vi "公式复合写入.vi"(8 "公式":cluster{"X^2":dbl, "X":dbl, "b":dbl}, 9 "量程下拉列表":enum16{"低量程", "高量程"}(ring), 10 "测量模式下拉列表":enum16{"水样测量", "零点核查", "跨度核查", "标样核查", "加标回收"}(ring), 11 "参数下拉列表":enum16{"COD", "氨氮", "总氮", "总磷"}(ring)) -> (3 "模型复制":T1)   [LabVIEW 2016, in "斯坦道氨氮.lvlib"]
uses:
  <vilib>/Utility/miscctls.llb/LVPointTypeDef.ctl
panel:
  out "连接的字符串":string
  in  "取消":bool
  in  "确认":bool
  in  "加标回收":bool
  in  "标样核查":bool
  in  "跨度核查":bool
  in  "空白核查":bool
  in  "水样测量":bool=TRUE
  # "请选择要写入的参数"
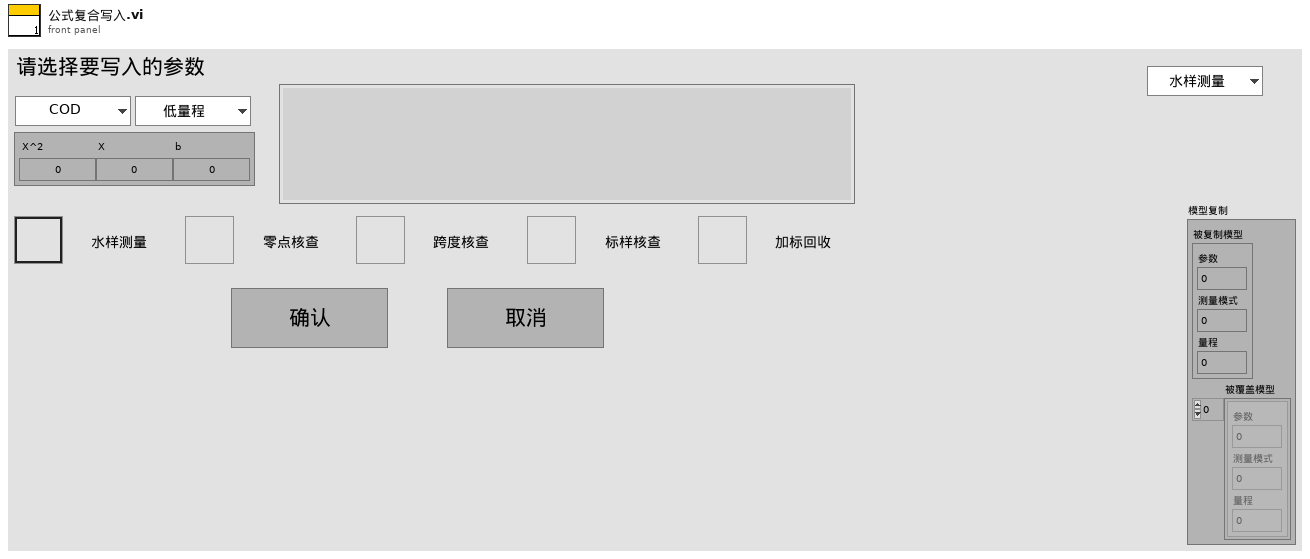
[diagram p1: front panel]
types:
  T1 = cluster{"被复制模型":cluster{"参数":u8, "测量模式":u8, "量程":u8}, "被覆盖模型":cluster{"参数":u8, "测量模式":u8, "量程":u8}[]}
  T2 = typedef "LVPointTypeDef.ctl" = cluster{"Horizontal":i16, "Vertical":i16}
  T3 = cluster{"COD":bool, "氨氮":bool, "总氮":bool, "总磷":bool}
  T4 = cluster{"测量量程":dbl, "测量精度":dbl, "测量间隔":dbl, "消解温度":dbl, "消解时长":dbl, "空白校准时间":timestamp, "曲线截距":dbl, "曲线斜率":dbl, "测量检出限":dbl, "测量信号值":dbl, "线性相关系数":dbl, "二次多项式系数":dbl, "标样校准时间":timestamp, "稀释倍数":dbl, "三项式系数":dbl, "空白标定系数":dbl, "量程系数":dbl, "F0/ORPA":dbl, "F1/ORPB":dbl, "F2/ORPK":dbl, "F3":dbl, "F4":dbl, "F5":dbl, "F6":dbl, "F7":dbl, "X0/滴定数":dbl, "量程":dbl}
  T5 = cluster{"参数下拉列表":enum16{"COD", "氨氮", "总氮", "总磷"}, "测量模式":enum16{"水样测量", "零点核查", "跨度核查", "标样核查", "加标回收"}, "量程下拉列表":enum16{"低量程", "高量程"}}
  T6 = cluster{"参数下拉列表":enum16{"COD", "氨氮", "总氮", "总磷"}, "测量模式":enum16{"水样测量", "零点核查", "跨度核查", "标样核查", "加标回收"}, "量程下拉列表":enum16{"低量程", "高量程"}}[]
  T7 = cluster{"参数下拉列表":enum16{"COD", "氨氮", "总氮", "总磷"}, "测量模式下拉列表":enum16{"水样测量", "零点核查", "跨度核查", "标样核查", "加标回收"}, "量程下拉列表":enum16{"低量程", "高量程"}}
  T8 = cluster{cluster{"参数下拉列表":enum16{"COD", "氨氮", "总氮", "总磷"}, "测量模式下拉列表":enum16{"水样测量", "零点核查", "跨度核查", "标样核查", "加标回收"}, "量程下拉列表":enum16{"低量程", "高量程"}}, cluster{"参数下拉列表":enum16{"COD", "氨氮", "总氮", "总磷"}, "测量模式下拉列表":enum16{"水样测量", "零点核查", "跨度核查", "标样核查", "加标回收"}, "量程下拉列表":enum16{"低量程", "高量程"}}[]}
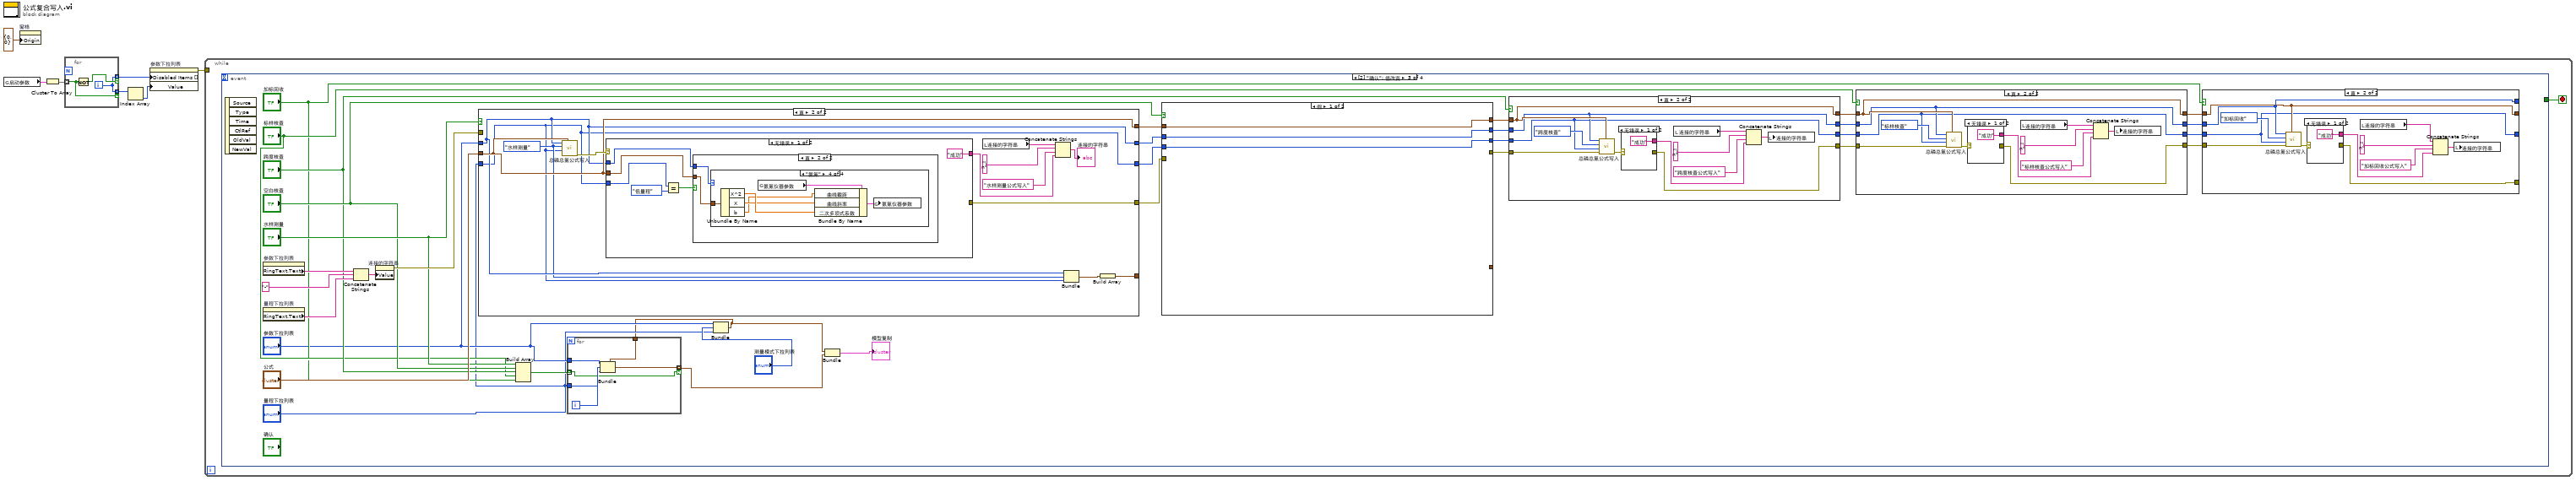
[diagram p0: block diagram]
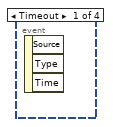
[diagram p2: hidden frame]
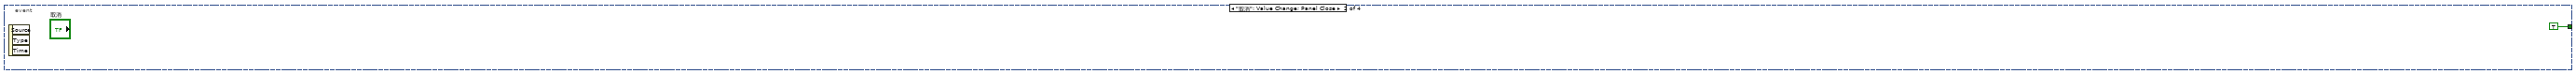
[diagram p3: hidden frame]
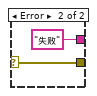
[diagram p5: hidden frame]
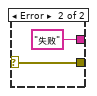
[diagram p7: hidden frame]
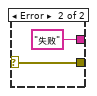
[diagram p9: hidden frame]
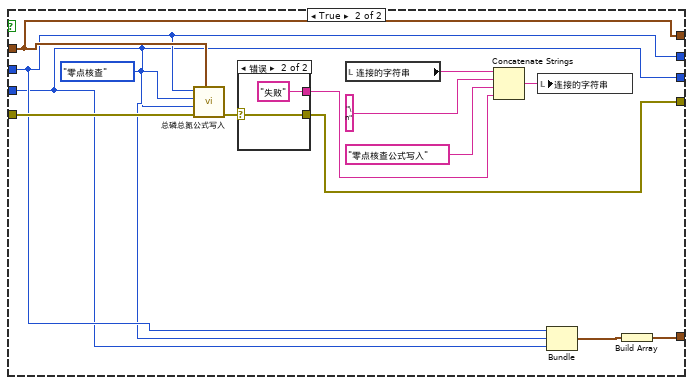
[diagram p10: hidden frame]
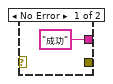
[diagram p11: hidden frame]
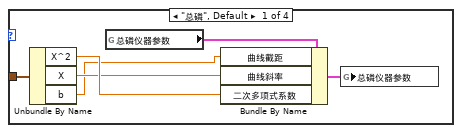
[diagram p14: hidden frame]
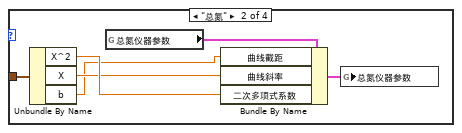
[diagram p15: hidden frame]
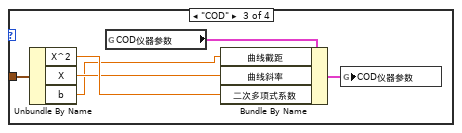
[diagram p16: hidden frame]
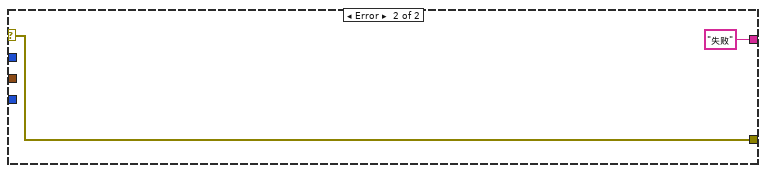
[diagram p17: hidden frame]
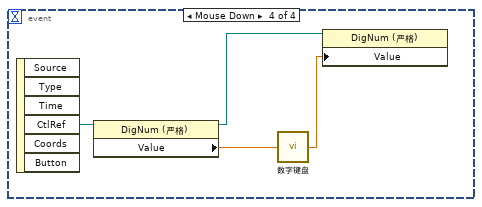
[diagram p18: hidden frame]
diagram:
  n1 = global read "总磷总氮断电保存全局变量.vi" "启动参数"() -> (w6:T3)
  n2 = property on="窗格" class="Pane"("Origin"=T2 {"Horizontal"=0, "Vertical"=0} ("原点")) -> ()  [unwired: 2 in, 2 out]
  n3 = Cluster To Array(cluster=w6) -> (array=w5:bool[])
  n4 = for {
    tunnel: w5 -> [w8] mode=indexing
    tunnel: [w9] -> w4 mode=indexing if=w10
    tunnel: [w9] -> w3 mode=indexing if=w8
    i -> [w9]
    n5 = Not(x=w8) -> (.not. x?=w10:bool)
  }
  n6 = Index Array(array=w3) -> (element=w2:i32)  [unwired: 1 in]
  n7 = property on="参数下拉列表" class="Enum (严格)"("Disabled Items []"=w4, "Value"=w2) -> (error out=w1:errorcluster)  [unwired: 2 in, 1 out]
  n8 = while {
    tunnel: w1 -> [_]
    stop <- w11 stop-if-true
    n9 = event shown="[2] \"确认\": 值改变" {
      selector: _ -> [_ _ _ _]
      dyn-events: _ -> [_ _ _ _]
      timeout: _ -> [_ _ _ _]
      tunnel: [_ TRUE _ _] -> w11
      event Timeout {
        n10 = event-data() -> ()  [unwired: 1 in, 3 out]
      }
      event "取消": Value Change; Panel Close {
        n11 = event-data() -> ()  [unwired: 1 in, 3 out]
      }
      event "确认": Value Change {
        n12 = event-data() -> ()  [unwired: 1 in, 6 out]
        n13 = property on="参数下拉列表" class="Enum (严格)"() -> ("RingText.Text"=w27:string)  [unwired: 2 in, 2 out]
        n14 = property on="量程下拉列表" class="Enum (严格)"() -> ("RingText.Text"=w26:string)  [unwired: 2 in, 2 out]
        n15 = Concatenate Strings(w27, "-" ("字符串"), w26) -> (w28:string)
        n16 = property on="连接的字符串" class="Str"("Value"=w28) -> (error out=w29:errorcluster)  [unwired: 2 in, 1 out]
        n17 = case shown="真" "水样测量" {
          tunnel: "公式" -> [w129 w135]
          tunnel: "参数下拉列表" -> [w128 w134]
          tunnel: "量程下拉列表" -> [w127 w132]
          tunnel: [w129 w135] -> w45
          tunnel: [w128 w134] -> w44
          tunnel: [w127 w132] -> w43
          tunnel: [_ w141] -> w31
          tunnel: w29 -> [_ _]
          tunnel: [_ w130] -> _
          frame False {
          }
          frame True {
            w133 = enum16{"水样测量", "零点核查", "跨度核查", "标样核查", "加标回收"}."水样测量" ("测量模式")
            n18 = call "总磷总氮公式写入.vi"("公式"=w135, "量程"=w132, "测量模式"=w133, "测量参数"=w134) -> ("error out"=w142:errorcluster)  [unwired: 7 in]
            n19 = case shown="无错误" w142 {
              selector: w142 -> [_ w176]
              tunnel: [_ w176] -> w141
              tunnel: ["成功" "失败"] -> w140
              tunnel: w132 -> [w147 _]
              tunnel: w134 -> [w144 _]
              tunnel: w135 -> [w143 _]
              frame No Error {
                n20 = Equal?(x=w147, y=enum16{"低量程", "高量程"}."低量程") -> (x = y?=w145:bool)
                n21 = case shown="真" w145 {
                  tunnel: w144 -> [_ w150]
                  tunnel: w143 -> [_ w149]
                  frame False {
                  }
                  frame True {
                    n22 = case shown="\"氨氮\"" w150 {
                      tunnel: w149 -> [w151 w157 w163 w169]
                      frame "总磷", Default {
                        n23 = Unbundle By Name(w151) -> ("X^2"=w154:dbl, "X"=w153:dbl, "b"=w152:dbl)
                        n24 = global read "总磷总氮断电保存全局变量.vi" "总磷仪器参数"() -> (w155:T4)
                        n25 = Bundle By Name(cluster=w155, "曲线截距"=w152, "曲线斜率"=w153, "二次多项式系数"=w154) -> (w156:T4)
                        n26 = global write "总磷总氮断电保存全局变量.vi" "总磷仪器参数"(w156) -> ()
                      }
                      frame "总氮" {
                        n27 = Unbundle By Name(w157) -> ("X^2"=w160:dbl, "X"=w159:dbl, "b"=w158:dbl)
                        n28 = global read "总磷总氮断电保存全局变量.vi" "总氮仪器参数"() -> (w161:T4)
                        n29 = Bundle By Name(cluster=w161, "曲线截距"=w158, "曲线斜率"=w159, "二次多项式系数"=w160) -> (w162:T4)
                        n30 = global write "总磷总氮断电保存全局变量.vi" "总氮仪器参数"(w162) -> ()
                      }
                      frame "COD" {
                        n31 = Unbundle By Name(w163) -> ("X^2"=w166:dbl, "X"=w165:dbl, "b"=w164:dbl)
                        n32 = global read "总磷总氮断电保存全局变量.vi" "COD仪器参数"() -> (w167:T4)
                        n33 = Bundle By Name(cluster=w167, "曲线截距"=w164, "曲线斜率"=w165, "二次多项式系数"=w166) -> (w168:T4)
                        n34 = global write "总磷总氮断电保存全局变量.vi" "COD仪器参数"(w168) -> ()
                      }
                      frame "氨氮" {
                        n35 = Unbundle By Name(w169) -> ("X^2"=w172:dbl, "X"=w171:dbl, "b"=w170:dbl)
                        n36 = global read "总磷总氮断电保存全局变量.vi" "氨氮仪器参数"() -> (w173:T4)
                        n37 = Bundle By Name(cluster=w173, "曲线截距"=w170, "曲线斜率"=w171, "二次多项式系数"=w172) -> (w174:T4)
                        n38 = global write "总磷总氮断电保存全局变量.vi" "氨氮仪器参数"(w174) -> ()
                      }
                    }
                  }
                }
              }
              frame Error {
              }
            }
            n39 = local read "连接的字符串"() -> (w137:string)
            n40 = Concatenate Strings(w137, "\n" ("字符串"), "水样测量公式写入", w140) -> (→"连接的字符串":string)
            n41 = Bundle("参数下拉列表"=w134, "测量模式"=w133, "量程下拉列表"=w132) -> (w131:T5)  [unwired: 1 in]
            n42 = Build Array(w131) -> (w130:T6)
          }
        }
        n43 = Build Array("水样测量", "空白核查", "跨度核查", "标样核查", "加标回收") -> (w19:bool[])
        n44 = Bundle("参数下拉列表"="参数下拉列表", "测量模式下拉列表"="测量模式下拉列表", "量程下拉列表"="量程下拉列表") -> (w15:T7)  [unwired: 1 in]
        n45 = for {
          tunnel: w19 -> [w48] mode=indexing
          tunnel: "参数下拉列表" -> [w52]
          tunnel: "量程下拉列表" -> [w50]
          tunnel: [w49] -> w14 mode=indexing if=w48
          tunnel: w15 -> [w47]
          i -> [w51]
          n46 = Bundle(cluster=w47, "参数下拉列表"=w52, "测量模式下拉列表"=w51, "量程下拉列表"=w50) -> (w49:T7)
        }
        n47 = Bundle(w15, w14) -> (→"模型复制":T8)  [unwired: 1 in]
        n48 = case shown="假" "空白核查" {
          tunnel: w45 -> [w109 w123]
          tunnel: w44 -> [w108 w113]
          tunnel: w43 -> [w107 w111]
          tunnel: [_ w118] -> w42
          tunnel: [w109 w123] -> w41
          tunnel: [w108 w113] -> w40
          tunnel: [w107 w111] -> w39
          tunnel: w31 -> [_ w122]
          tunnel: [_ w110] -> _
          frame False {
          }
          frame True {
            w112 = enum16{"水样测量", "零点核查", "跨度核查", "标样核查", "加标回收"}."零点核查" ("测量模式")
            n49 = call "总磷总氮公式写入.vi"("公式"=w123, "error in (no error)"=w122, "量程"=w111, "测量模式"=w112, "测量参数"=w113) -> ("error out"=w119:errorcluster)  [unwired: 6 in]
            n50 = case shown="错误" w119 {
              selector: w119 -> [_ w126]
              tunnel: [_ w126] -> w118
              tunnel: ["成功" "失败"] -> w120
              frame No Error {
              }
              frame Error {
              }
            }
            n51 = local read "连接的字符串"() -> (w117:string)
            n52 = Concatenate Strings(w117, "\n" ("字符串"), "零点核查公式写入", w120) -> (w115:string)
            n53 = local write "连接的字符串"(w115) -> ()
            n54 = Bundle("参数下拉列表"=w113, "测量模式"=w112, "量程下拉列表"=w111) -> (w114:T5)  [unwired: 1 in]
            n55 = Build Array(w114) -> (w110:T6)
          }
        }
        n56 = case shown="真" "跨度核查" {
          tunnel: w41 -> [w91 w102]
          tunnel: w40 -> [w90 w101]
          tunnel: w39 -> [w89 w100]
          tunnel: [w91 w102] -> w38
          tunnel: [w90 w101] -> w36
          tunnel: [w89 w100] -> w35
          tunnel: w42 -> [_ w99]
          tunnel: [_ w92] -> w30
          frame False {
          }
          frame True {
            n57 = call "总磷总氮公式写入.vi"("公式"=w102, "error in (no error)"=w99, "量程"=w100, "测量模式"=enum16{"水样测量", "零点核查", "跨度核查", "标样核查", "加标回收"}."跨度核查", "测量参数"=w101) -> ("error out"=w93:errorcluster)  [unwired: 6 in]
            n58 = case shown="无错误" w93 {
              selector: w93 -> [_ w106]
              tunnel: [_ w106] -> w92
              tunnel: ["成功" "失败"] -> w94
              frame No Error {
              }
              frame Error {
              }
            }
            n59 = local read "连接的字符串"() -> (w96:string)
            n60 = Concatenate Strings(w96, "\n" ("字符串"), "跨度核查公式写入", w94) -> (w98:string)
            n61 = local write "连接的字符串"(w98) -> ()
          }
        }
        n62 = case shown="真" "标样核查" {
          tunnel: w38 -> [w73 w84]
          tunnel: w36 -> [w72 w83]
          tunnel: w35 -> [w71 w82]
          tunnel: [_ w74] -> w32
          tunnel: [w73 w84] -> w37
          tunnel: [w72 w83] -> w34
          tunnel: [w71 w82] -> w33
          tunnel: w30 -> [_ w81]
          frame False {
          }
          frame True {
            n63 = call "总磷总氮公式写入.vi"("公式"=w84, "error in (no error)"=w81, "量程"=w82, "测量模式"=enum16{"水样测量", "零点核查", "跨度核查", "标样核查", "加标回收"}."标样核查", "测量参数"=w83) -> ("error out"=w75:errorcluster)  [unwired: 6 in]
            n64 = case shown="无错误" w75 {
              selector: w75 -> [_ w88]
              tunnel: [_ w88] -> w74
              tunnel: ["成功" "失败"] -> w76
              frame No Error {
              }
              frame Error {
              }
            }
            n65 = local read "连接的字符串"() -> (w78:string)
            n66 = Concatenate Strings(w78, "\n" ("字符串"), "标样核查公式写入", w76) -> (w80:string)
            n67 = local write "连接的字符串"(w80) -> ()
          }
        }
        n68 = case shown="真" "加标回收" {
          tunnel: w37 -> [w55 w66]
          tunnel: w34 -> [w54 w65]
          tunnel: w33 -> [w53 w64]
          tunnel: [w55 w66] -> _
          tunnel: [w54 w65] -> _
          tunnel: [w53 w64] -> _
          tunnel: w32 -> [_ w63]
          tunnel: [_ w56] -> _
          frame False {
          }
          frame True {
            n69 = call "总磷总氮公式写入.vi"("公式"=w66, "error in (no error)"=w63, "量程"=w64, "测量模式"=enum16{"水样测量", "零点核查", "跨度核查", "标样核查", "加标回收"}."加标回收", "测量参数"=w65) -> ("error out"=w57:errorcluster)  [unwired: 6 in]
            n70 = case shown="无错误" w57 {
              selector: w57 -> [_ w70]
              tunnel: [_ w70] -> w56
              tunnel: ["成功" "失败"] -> w58
              frame No Error {
              }
              frame Error {
              }
            }
            n71 = local read "连接的字符串"() -> (w60:string)
            n72 = Concatenate Strings(w60, "\n" ("字符串"), "加标回收公式写入", w58) -> (w62:string)
            n73 = local write "连接的字符串"(w62) -> ()
          }
        }
      }
      event "公式.X^2", "公式.X", "公式.b": Mouse Down {
        n74 = event-data() -> ("CtlRef"=w180:refnum<vi>)  [unwired: 1 in, 5 out]
        n75 = property class="DigNum (严格)"(reference=w180) -> (reference out=w177:refnum<vi>, "Value"=w179:dbl)  [unwired: 1 in, 1 out]
        n76 = call "数字键盘.vi"("OldNumber"=w179) -> ("NewNumber"=w178:dbl)
        n77 = property class="DigNum (严格)"(reference=w177, "Value"=w178) -> ()  [unwired: 1 in, 2 out]
      }
    }
  }
